vi "Clip Waveform.vi"(0 "signal configuration":refnum<class "SV Signal.lvclass">, 5 "input waveform":waveform(dbl), 11 "error in (no error)":errorcluster) -> (4 "signal configuration":refnum<class "SV Signal.lvclass">, 6 "offset waveform":waveform(dbl), 15 "error out":errorcluster)   [LabVIEW 2017, in "SV Signal.lvclass"]
uses:
  <vilib>/addons/_NISVFA/_Generation/Signal Generation/SV Signal/SV Signal.lvclass
  <vilib>/addons/_NISVFA/_Generation/Signal Generation/SV Signal/SV Signal.lvclass/SV Signal.ctl
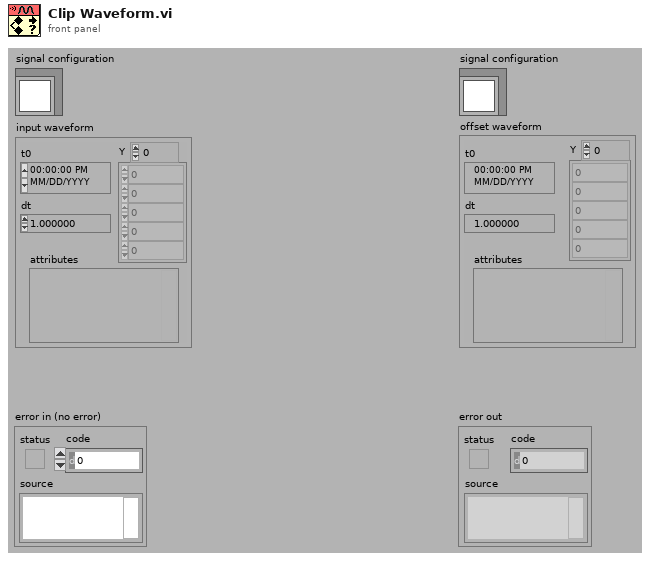
[diagram p1: front panel]
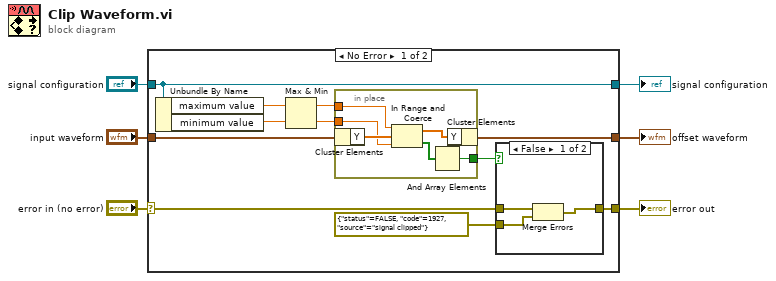
[diagram p0: block diagram]
diagram:
  n1 = case shown="No Error" "error in (no error)" {
    selector: "error in (no error)" -> [w9 w29]
    tunnel: [w8 w29] -> w5
    tunnel: [w17 w30] -> w3
    tunnel: "signal configuration" -> [w17 w30]
    tunnel: "input waveform" -> [w16 w28]
    tunnel: [w15 w28] -> w1
    frame No Error {
      n2 = Unbundle By Name(w17) -> ("maximum value"=w11:dbl, "minimum value"=w14:dbl)
      n3 = Max & Min(x=w11, y=w14) -> (max(x,y)=w13:dbl, min(x,y)=w12:dbl)
      n4 = in-place {
        in-place-border: w13 -> [w26]
        in-place-border: w12 -> [w25]
        in-place-border: [w23] -> w10
        n5 = in-place-cluster #1(w16) -> ("Y"=w27:dbl[])
        n6 = In Range and Coerce(upper limit=w26, x=w27, lower limit=w25) -> (coerced(x)=w24:dbl[], In Range?=w22:bool[])
        n7 = And Array Elements(Boolean array=w22) -> (logical AND=w23:bool)
        n8 = in-place-cluster #1("Y"=w24) -> (w15:waveform(dbl))
      }
      n9 = case shown="False" w10 {
        tunnel: w9 -> [w20 w21]
        tunnel: [w18 w21] -> w8
        tunnel: errorcluster {"status"=FALSE, "code"=1927, "source"="signal clipped"} ("error IO") -> [w19 _]
        frame False {
          n10 = Merge Errors(w20, w19) -> (w18:errorcluster)
        }
        frame True {
        }
      }
    }
    frame Error {
    }
  }
  "error out" <- w5
  "signal configuration" <- w3
  "offset waveform" <- w1
